vi "myRIO_BRig_Host_formatData_getHeaders_dataExp.vi"() -> (3 "output_stringArray_dataExp":string[](array[string]))   [LabVIEW 2014]
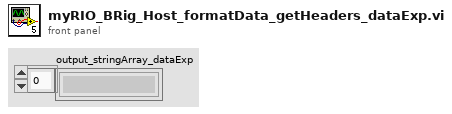
[diagram p1: front panel]
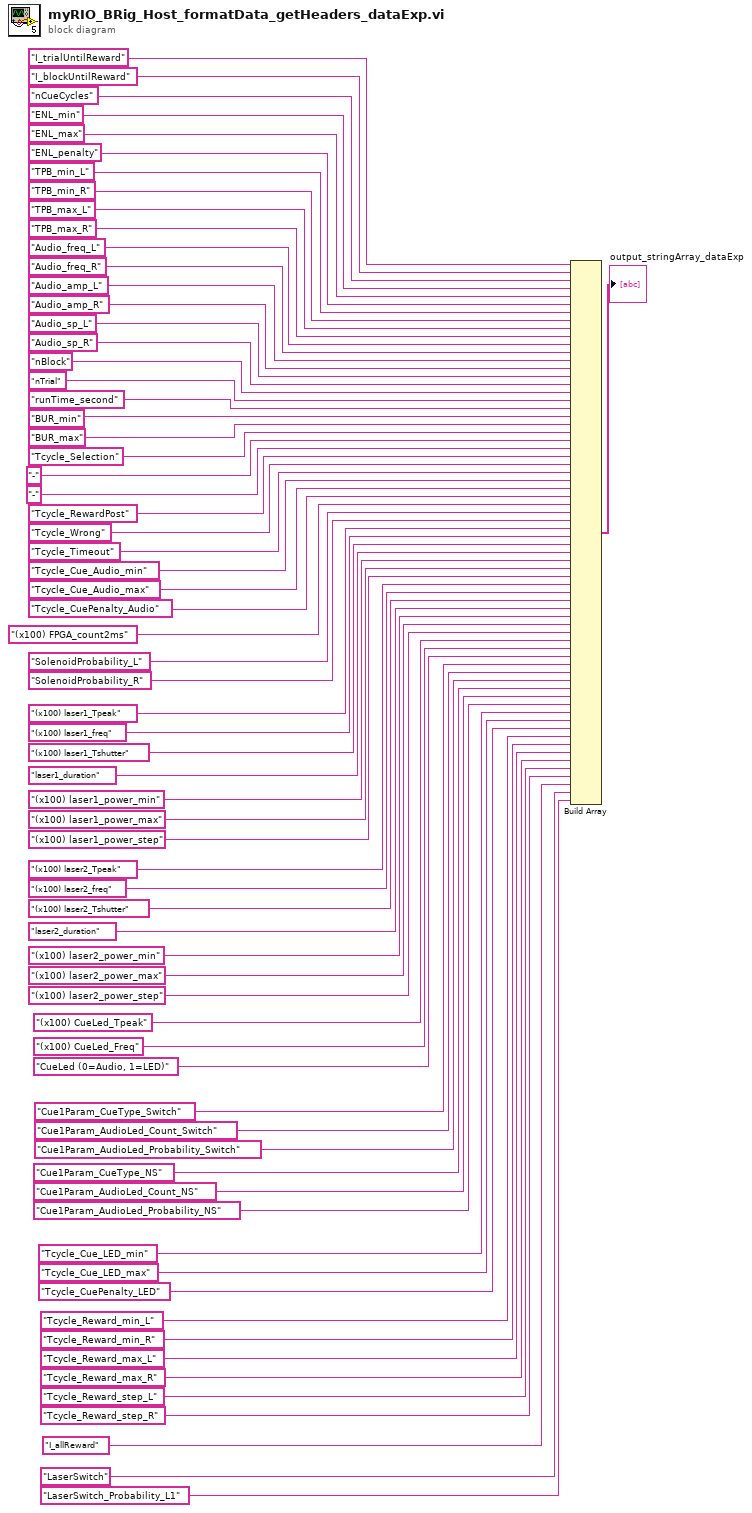
[diagram p0: block diagram]
diagram:
  n1 = Build Array("I_trialUntilReward", "I_blockUntilReward", "nCueCycles", "ENL_min", "ENL_max", "ENL_penalty", "TPB_min_L", "TPB_min_R", "TPB_max_L", "TPB_max_R", "Audio_freq_L", "Audio_freq_R", "Audio_amp_L", "Audio_amp_R", "Audio_sp_L", "Audio_sp_R", "nBlock", "nTrial", "runTime_second", "BUR_min", "BUR_max", "Tcycle_Selection", "-", "-", "Tcycle_RewardPost", "Tcycle_Wrong", "Tcycle_Timeout", "Tcycle_Cue_Audio_min", "Tcycle_Cue_Audio_max", "Tcycle_CuePenalty_Audio", "(x100) FPGA_count2ms", "SolenoidProbability_L", "SolenoidProbability_R", "(x100) laser1_Tpeak", "(x100) laser1_freq", "(x100) laser1_Tshutter", "laser1_duration", "(x100) laser1_power_min", "(x100) laser1_power_max", "(x100) laser1_power_step", "(x100) laser2_Tpeak", "(x100) laser2_freq", "(x100) laser2_Tshutter", "laser2_duration", "(x100) laser2_power_min", "(x100) laser2_power_max", "(x100) laser2_power_step", "(x100) CueLed_Tpeak", "(x100) CueLed_Freq", "CueLed (0=Audio, 1=LED)", "Cue1Param_CueType_Switch", "Cue1Param_AudioLed_Count_Switch", "Cue1Param_AudioLed_Probability_Switch", "Cue1Param_CueType_NS", "Cue1Param_AudioLed_Count_NS", "Cue1Param_AudioLed_Probability_NS", "Tcycle_Cue_LED_min", "Tcycle_Cue_LED_max", "Tcycle_CuePenalty_LED", "Tcycle_Reward_min_L", "Tcycle_Reward_min_R", "Tcycle_Reward_max_L", "Tcycle_Reward_max_R", "Tcycle_Reward_step_L", "Tcycle_Reward_step_R", "I_allReward", "LaserSwitch", "LaserSwitch_Probability_L1") -> (→"output_stringArray_dataExp":string[])
